vi "TDMS File Split.vi"(0 "serial input channel":string="SI0", 5 "tdms file directory":path, 7 "progress ref":refnum<vi>, 11 "error in":errorcluster) -> (15 "error out":errorcluster)   [LabVIEW 2023, in "GettingStarted_Common_148X_Host.lvlib"]
uses:
  GettingStarted_Common_148X_Host.lvlib
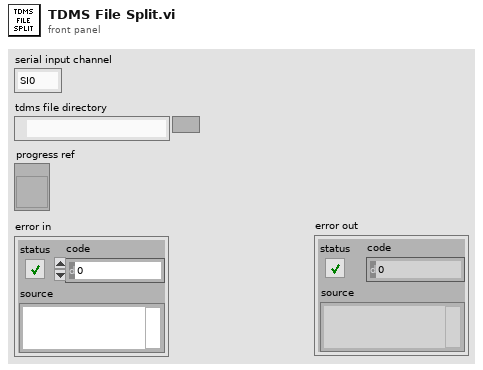
[diagram p1: front panel]
types:
  T1 = enum16{"open", "open or create", "create or replace", "create", "open (read-only)"}
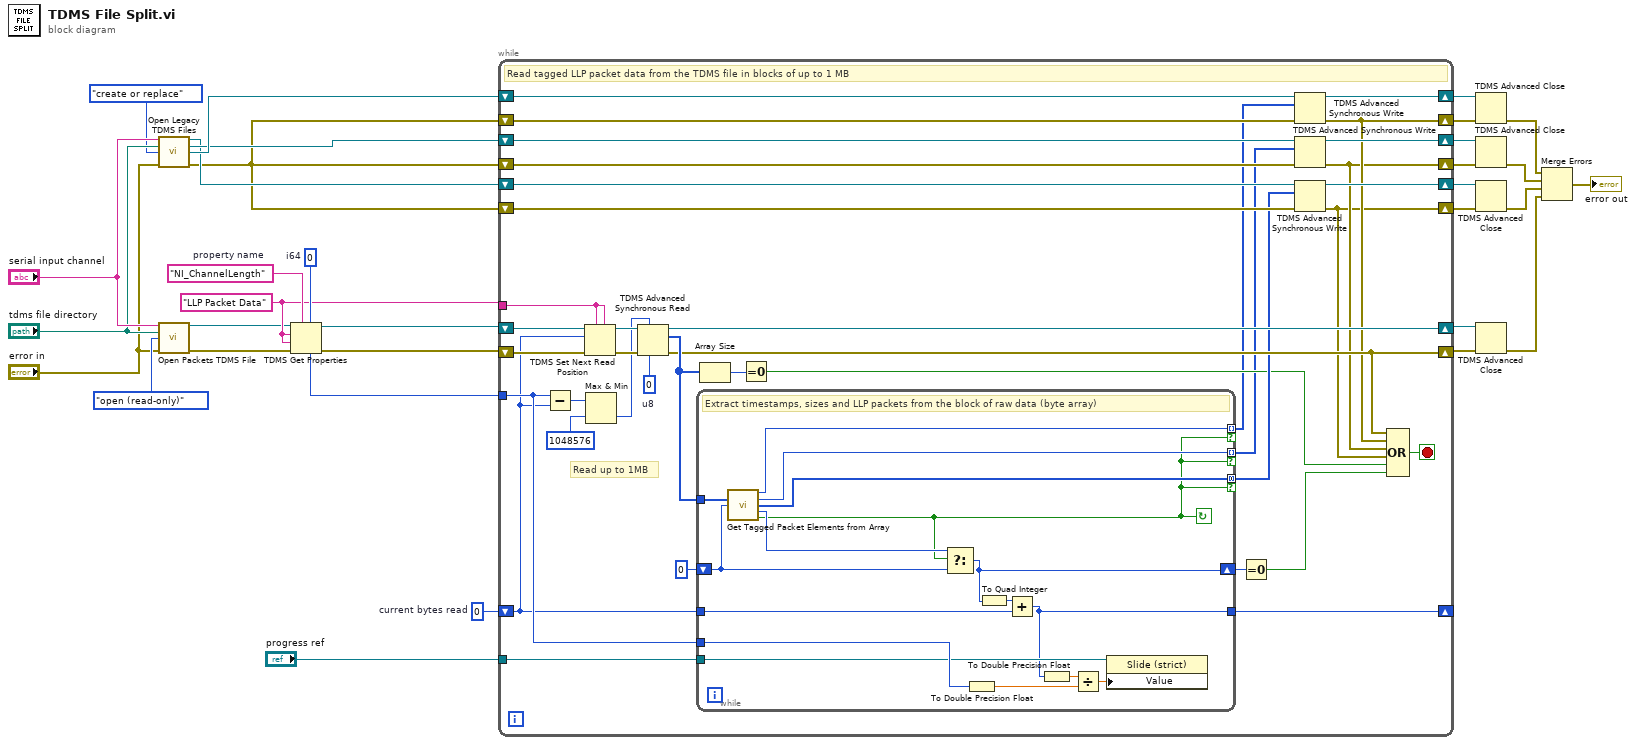
[diagram p0: block diagram]
diagram:
  w1 = i64 0  # current bytes read
  w30 = i64 0  # i64
  w31 = "NI_ChannelLength"  # property name
  w27 = "LLP Packet Data" ("channel and group name")
  n1 = call "Open Legacy TDMS Files.vi"("serial input channel"="serial input channel", "base tdms file path"="tdms file directory", "file operation type"=T1."create or replace", "error in (no error)"="error in") -> ("data file ref"=w12:refnum<k34>, "sizes file ref"=w13:refnum<k34>, "timestamp file ref"=w14:refnum<k34>, "error out"=w11:errorcluster)  [unwired: 8 in]
  n2 = call "Open Packets TDMS File.vi"("serial input channel"="serial input channel", "base tdms file path"="tdms file directory", "file operation type"=T1."open (read-only)", "error in"="error in") -> ("packets file ref"=w2:refnum<k34>, "error out"=w3:errorcluster)  [unwired: 10 in]
  n3 = TDMS Get Properties(5:w30, 7:w31, 8:w3, 9:w27, 10:w27, 11:w2) -> (0:w29:errorcluster, 3:w28:refnum<k34>, 4:w17:i64)  [unwired: 3 out]
  n4 = while {
    shift-right: [w52] -> w22
    shift-left: w29 -> [w68]
    shift-right: [w59] -> w23
    shift-left: w28 -> [w67]
    shift-right: [w53] -> _
    shift-left: w1 -> [w54]
    tunnel: w17 -> [w56]
    tunnel: w27 -> [w60]
    tunnel: "progress ref" -> [w57]
    shift-right: [w51] -> w6
    shift-left: w14 -> [w47]
    shift-right: [w41] -> w5
    shift-left: w11 -> [w48]
    shift-right: [w50] -> w7
    shift-left: w13 -> [w46]
    shift-right: [w40] -> w8
    shift-left: w11 -> [w45]
    shift-right: [w49] -> w9
    shift-left: w12 -> [w44]
    shift-right: [w39] -> w10
    shift-left: w11 -> [w43]
    stop <- w64 stop-if-true
    w69 = u8 0  # u8
    # "Read up to 1MB"
    # "Read tagged LLP packet data from the TDMS file in blocks of up to 1 MB"
    n5 = Subtract(x=w56, y=w54) -> (x-y=w62:i64)
    n6 = TDMS Set Next Read Position(5:w60, 7:w60, 8:w68, 10:w54, 11:w67) -> (0:w65:errorcluster, 3:w66:refnum<k34>)  [unwired: 1 in]
    n7 = Max & Min(x=w62, y=i64 1048576 ("max bytes to read per iteration")) -> (min(x,y)=w61:i64)  [unwired: 1 out]
    n8 = TDMS Advanced Synchronous Read(6:w69, 7:w61, 8:w65, 11:w66) -> (0:w52:errorcluster, 2:w58:u8[], 3:w59:refnum<k34>)  [unwired: 1 out]
    n9 = while {
      tunnel: w58 -> [w84]
      shift-right: [w74] -> w35
      shift-left: u32 0 ("total tagged packet size (bytes)") -> [w83]
      tunnel: w56 -> [w79]
      tunnel: w57 -> [w78]
      tunnel: w54 -> [w77]
      tunnel: [w76] -> w53
      tunnel: [w73] -> w42 mode=concatenating if=w70
      tunnel: [w72] -> w34 mode=indexing if=w70
      tunnel: [w71] -> w33 mode=indexing if=w70
      stop <- w70 continue-if-true
      # "Extract timestamps, sizes and LLP packets from the block of raw data (byte array)"
      n10 = call "Get Tagged Packet Elements from Array.vi"("tagged packet data in"=w84, "tagged packet offset"=w83) -> ("packet timestamp"=w71:u64, "packet data length (bytes)"=w72:u32, "packet data"=w73:u8[], "total tagged packet size (bytes)"=w85:u32, "valid packet data?"=w70:bool)  [unwired: 9 in]
      n11 = Select(t=w85, s=w70, f=w83) -> (s? t:f=w74:u32)
      n12 = To Double Precision Float(number=w79) -> (double precision float=w81:dbl)
      n13 = To Quad Integer(1:w74) -> (0:w75:i64)
      n14 = Add(x=w75, y=w77) -> (x+y=w76:i64)
      n15 = To Double Precision Float(number=w76) -> (double precision float=w80:dbl)
      n16 = Divide(x=w80, y=w81) -> (x/y=w82:dbl)
      n17 = property class="Slide (strict)"(reference=w78, "Value"=w82) -> ()  [unwired: 1 in, 2 out]
    }
    n18 = Array Size(array=w58) -> (size(s)=w63:i32)
    n19 = Equal To 0?(x=w63) -> (x = 0?=w38:bool)
    n20 = Equal To 0?(x=w35) -> (x = 0?=w37:bool)
    n21 = TDMS Advanced Synchronous Write(8:w48, 10:w33, 11:w47) -> (0:w41:errorcluster, 3:w51:refnum<k34>)
    n22 = TDMS Advanced Synchronous Write(8:w45, 10:w34, 11:w46) -> (0:w40:errorcluster, 3:w50:refnum<k34>)
    n23 = TDMS Advanced Synchronous Write(8:w43, 10:w42, 11:w44) -> (0:w39:errorcluster, 3:w49:refnum<k34>)
    n24 = Compound Arithmetic op=OR(w52, w41, w40, w39, w38, w37) -> (w64:bool)
  }
  n25 = TDMS Advanced Close(8:w5, 11:w6) -> (0:w20:errorcluster)  [unwired: 2 in, 1 out]
  n26 = TDMS Advanced Close(8:w8, 11:w7) -> (0:w19:errorcluster)  [unwired: 2 in, 1 out]
  n27 = TDMS Advanced Close(8:w10, 11:w9) -> (0:w18:errorcluster)  [unwired: 2 in, 1 out]
  n28 = TDMS Advanced Close(8:w22, 11:w23) -> (0:w21:errorcluster)  [unwired: 2 in, 1 out]
  n29 = Merge Errors(w20, w19, w18, w21) -> (→"error out":errorcluster)
